vi "1B calc wind acceleration.vi"(9 "time elapsed since last iteration":dbl, 10 "Apparent Wind Speed in":T2, 11 "Apparent Wind\nDirection":T1) -> (3 "Wind dV":T2)   [LabVIEW 2011]
doc: "Calculates dV due to the wind.\nTODO: currently only does acceleration in the forward direction. should be upgraded to have a side force as well, which can be balanced by a hydrodynamic side force.\nTODO: make this depend on sail angle as well.\nCurrently uses a very simple algorithm: if the boat is within 35 degrees of the wind, it is in irons, and gets a small constant acceleration. Otherwise it gets acceleration proportional to the wind speed."
uses:
  2-Think/2 Typedefs/apparent wind speed.ctl
  2-Think/2 Typedefs/apparent wind direction.ctl
panel:
  out "In Irons?":bool
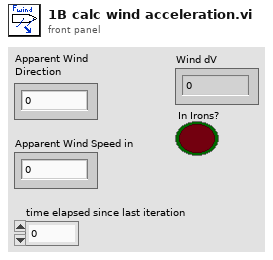
[diagram p1: front panel]
types:
  T1 = typedef "apparent wind direction.ctl" = dbl
  T2 = typedef "apparent wind speed.ctl" = dbl
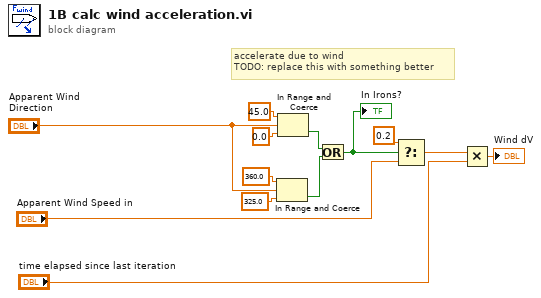
[diagram p0: block diagram]
diagram:
  # "accelerate due to wind\nTODO: replace this with something better"
  n1 = In Range and Coerce(upper limit=T1 360.0 ("lower limit"), x="Apparent Wind\nDirection", lower limit=T1 325.0) -> (In Range?=w8:bool)  [unwired: 1 out]
  n2 = In Range and Coerce(upper limit=T1 45.0 ("lower limit"), x="Apparent Wind\nDirection", lower limit=T1 0.0) -> (In Range?=w4:bool)  [unwired: 1 out]
  n3 = Or(x=w4, y=w8) -> (x .or. y?=w1:bool)
  "In Irons?" <- w1
  n4 = Select(t=T2 0.2 ("Apparent Wind Speed"), s=w1, f="Apparent Wind Speed in") -> (s? t:f=w12:T2)
  n5 = Multiply(x=w12, y="time elapsed since last iteration") -> (x*y=→"Wind dV":T2)
